vi "acende_led_comparacao.vi"() -> ()   [LabVIEW 2020]
panel:
  out "Se T > 35 C":bool
  in  "Termometro":dbl(slide) scale=0.0..100.0
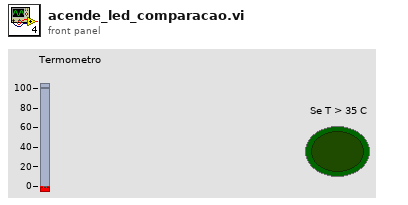
[diagram p1: front panel]
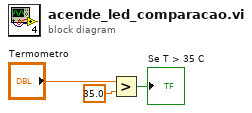
[diagram p0: block diagram]
diagram:
  n1 = Greater?(x="Termometro", y=35.0) -> (0:→"Se T > 35 C":bool)
